vi "Configuration 2.0 Finalize.vi"(8 "error in (no error)":errorcluster, 10 "file version (x.y)":T2, 11 "configuration 2.0":T1) -> (0 "error out":errorcluster, 2 "final file version":T2, 3 "configuration json":string)   [LabVIEW 2017, in "DSF Core.lvlib" / "Configuration Session.lvclass"]
uses:
  Configuration Session.lvclass
  Typedefs/DSF Version Info.ctl
  DSF Core.lvlib
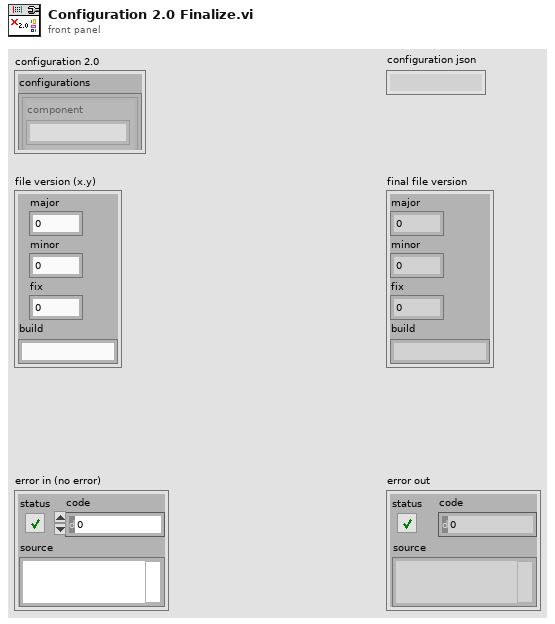
[diagram p1: front panel]
types:
  T1 = cluster{"configurations":cluster{"component":string, "data":string, "data version":cluster{"major":i32, "minor":i32, "fix":i32, "build":string}}[], "plugins":cluster{"configurations":cluster{"component":string, "data":string, "data version":cluster{"major":i32, "minor":i32, "fix":i32, "build":string}}[], "threads":cluster{"configurations":cluster{"component":string, "data":string, "data version":cluster{"major":i32, "minor":i32, "fix":i32, "build":string}}[], "groups":cluster{"configurations":cluster{"component":string, "data":string, "data version":cluster{"major":i32, "minor":i32, "fix":i32, "build":string}}[], "transfers":cluster{"configurations":cluster{"component":string, "data":string, "data version":cluster{"major":i32, "minor":i32, "fix":i32, "build":string}}[]}[]}[]}[]}[]}
  T2 = typedef "DSF Core.lvlib/DSF Version Info.ctl" = cluster{"major":i32, "minor":i32, "fix":i32, "build":string}
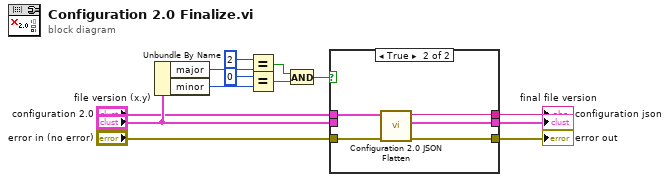
[diagram p0: block diagram]
diagram:
  n1 = Unbundle By Name("file version (x.y)") -> ("major"=w12:i32, "minor"=w13:i32)
  n2 = Equal?(x=2, y=w12) -> (x = y?=w8:bool)
  n3 = Equal?(x=0, y=w13) -> (x = y?=w9:bool)
  n4 = And(x=w8, y=w9) -> (x .and. y?=w7:bool)
  n5 = case shown="True" w7 {
    tunnel: "error in (no error)" -> [w14 w19]
    tunnel: "configuration 2.0" -> [_ w18]
    tunnel: [w14 w17] -> w4
    tunnel: "file version (x.y)" -> [_ _]
    tunnel: [_ w16] -> w5
    tunnel: [_ w15] -> w2
    frame False {
      # "2.0 is not backwards compatible."
    }
    frame True {
      n6 = call "Configuration 2.0 JSON Flatten.vi"("error in (no error)"=w19, "dsf configuration 2.0"=w18) -> ("error out"=w17:errorcluster, "dsf version"=w15:T2, "dsf configuration json"=w16:string)  [unwired: 7 in]
    }
  }
  "error out" <- w4
  "final file version" <- w2
  "configuration json" <- w5
